vi "Open Level Meter Device.vi"(8 "error in (no error)":errorcluster, 10 "Device Identifier":string, 11 "Mercury Reference In":T1) -> (0 "error out":errorcluster, 3 "Mercury Reference Out":T1)   [LabVIEW 2018, in "Mercury iXX.lvlib" / "Level Meter.lvlib"]
doc: "Opens the level meter device."
uses:
  Level Meter.lvlib
  Mercury Reference.ctl
  Comms Transport Layer.ctl
  Query Dynamic Reference.ctl
  System.lvlib
  Mercury iXX.lvlib
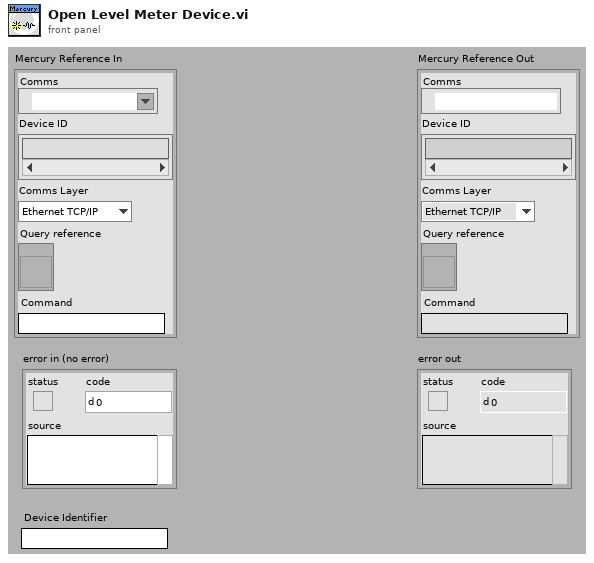
[diagram p1: front panel]
types:
  T1 = typedef "Mercury iXX.lvlib/Mercury Reference.ctl" = cluster{"Comms":refnum<visa-resource-name>, "Device ID":string[], "Comms Layer":T2, "Command":string, "Query reference":T3}
  T2 = typedef "Mercury iXX.lvlib/Comms Transport Layer.ctl" = enum16{"Ethernet TCP/IP", "USB", "ISOBus - RS-232", "GPIB"}
  T3 = typedef "Mercury iXX.lvlib/Query Dynamic Reference.ctl" = refnum<vi>
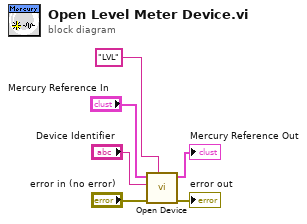
[diagram p0: block diagram]
diagram:
  n1 = call "Open Device.vi"("Device Type"="LVL", "error in (no error)"="error in (no error)", "Device Identifier"="Device Identifier", "Mercury Reference In"="Mercury Reference In") -> ("error out"=→"error out":errorcluster, "Mercury Reference Out"=→"Mercury Reference Out":T1)  [unwired: 6 out]
